vi "FM Ch Read Refresh Frm.vi"(6 "pReturned":u32, 7 "pBuffer":string, 9 "BufSize":u32, 10 "Channel":u8, 11 "devId":i32) -> (2 "devId out":i32, 3 "function return":u8, 4 "pReturned out":u32, 5 "pBuffer out":string)   [LabVIEW 2013, in "CHR34XXX.lvlib"]
doc: "DLL BOOL __stdcall CHR34XXX_FM_Ch_RxMode(IN int devId,IN BYTE Channel,IN BYTE RxMode); DLL BOOL __stdcall CHR34XXX_FM_Ch_RxFrmCount(IN int devId,IN BYTE Channel,OUT DWORD *FrmCnt); DLL BOOL __stdcall CHR34XXX_FM_Ch_ReadFrm(IN int devId,IN BYTE Channel,IN DWORD BufSize,OUT BYTE *pBuffer,OUT DWORD *pReturned); DLL BYTE __stdcall CHR34XXX_FM_Ch_ReadRefreshFrm(IN int devId,IN BYTE Channel,IN DWORD BufSize,OUT BYTE *pBuffer,OUT DWORD *pReturned);"
uses:
  CHR34XXX.lvlib
  CHR34XXX.dll
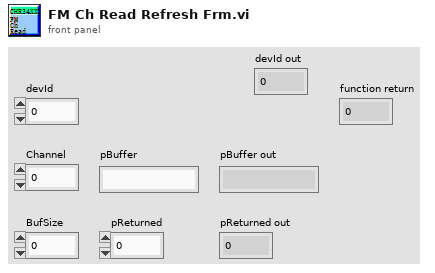
[diagram p1: front panel]
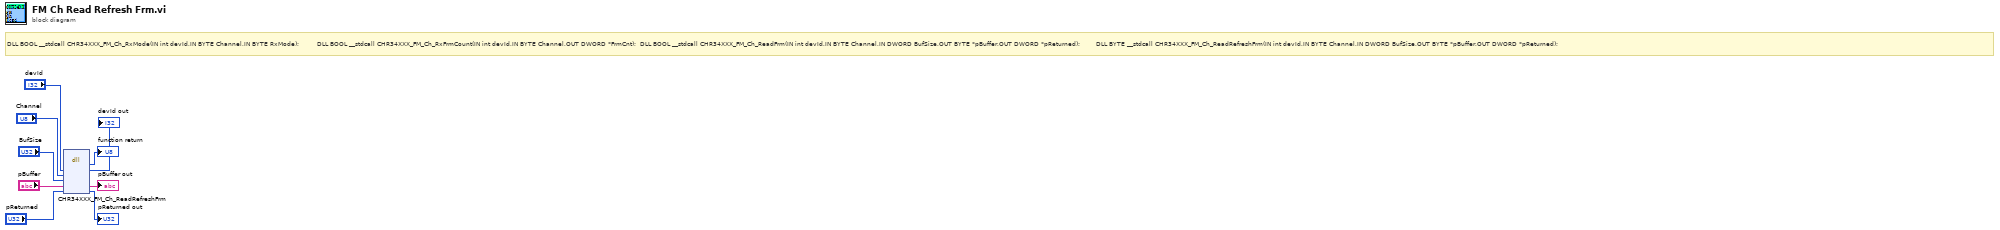
[diagram p0: block diagram]
diagram:
  # "DLL BOOL __stdcall CHR34XXX_FM_Ch_RxMode(IN int devId,IN BYTE Channel,IN BYTE RxMode);         DLL BOOL __stdcall CHR34XXX_FM_Ch_RxFrmCount(IN int devId,IN BYTE Channel,OUT DWORD *FrmCnt);  DLL BOOL __stdcall CHR34XXX_FM_Ch_ReadFrm(IN int devId,IN BYTE Channel,IN DWORD BufSize,OUT BYTE *pBuffer,OUT DWORD *pReturned);        DLL BYTE __stdcall CHR34XXX_FM_Ch_ReadRefreshFrm(IN int devId,IN BYTE Channel,IN DWORD BufSize,OUT BYTE *pBuffer,OUT DWORD *pReturned);"
  n1 = dll-call lib="C:/Users/Administrator/Desktop/CHR34XXX_lv/lv_lib/CHR34XXX.*" fn="CHR34XXX_FM_Ch_ReadRefreshFrm"("devId"="devId", "Channel"="Channel", "BufSize"="BufSize", "pBuffer"="pBuffer", "pReturned"="pReturned") -> (→"function return":u8, "devId"=→"devId out":i32, "pBuffer"=→"pBuffer out":string, "pReturned"=→"pReturned out":u32)  [unwired: 5 in, 2 out]
